vi "Get Node ID.vi"(10 "Node":variant, 11 "Abstract Graph in":refnum<class "Abstract Graph.lvclass">) -> (1 "Node Exist":bool, 2 "Node ID":string, 3 "Abstract Graph out":refnum<class "Abstract Graph.lvclass">)   [LabVIEW 2021, in "GraphLib.lvlib" / "Abstract Graph.lvclass"]
uses:
  Abstract Graph.lvclass
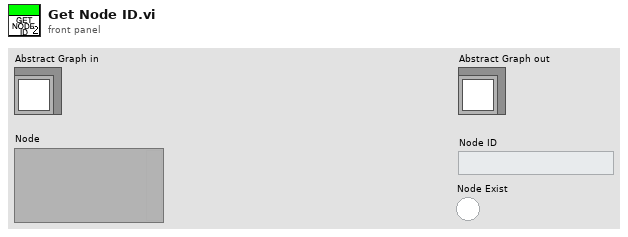
[diagram p1: front panel]
types:
  T1 = typedef "GraphLib.lvlib/Node Internal.ctl" = cluster{"Node":T2, "Edge IDs":set{string}}
  T2 = typedef "GraphLib.lvlib/Node.ctl" = cluster{"Value":variant, "Attributes":map{string, variant}}
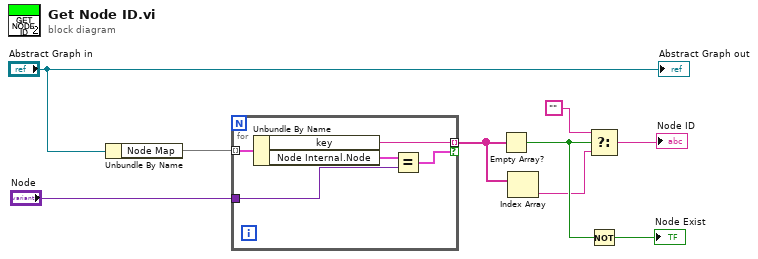
[diagram p0: block diagram]
diagram:
  n1 = Unbundle By Name("Abstract Graph in") -> ("Node Map"=w9:map{string, T1})
  n2 = for {
    tunnel: w9 -> [w14] mode=indexing
    tunnel: [w13] -> w7 mode=indexing if=w10
    tunnel: "Node" -> [w11]
    n3 = Unbundle By Name(w14) -> ("key"=w13:string, "Node Internal.Node"=w12:T2)
    n4 = Equal?(x=w12, y=w11) -> (x = y?=w10:cluster{"Value":bool, "Attributes":bool})
  }
  n5 = Empty Array?(array=w7) -> (empty?=w5:bool)
  n6 = Index Array(array=w7) -> (element=w1:string)  [unwired: 1 in]
  n7 = Select(t="", s=w5, f=w1) -> (s? t:f=→"Node ID":string)
  n8 = Not(x=w5) -> (.not. x?=→"Node Exist":bool)
  "Abstract Graph out" <- "Abstract Graph in"
